vi "Get_Kinect_Depth_Array.vi"(8 "Index":i32, 9 "Far_Clip_Plane":u16=2040, 11 "Refnum_in":T1=refnum) -> (0 "2D_Array":u16[][](array[numeric]), 1 "1D_Array":u16[](array[numeric]), 2 "Image_out":T1, 3 "Refnum_out":T1)   [LabVIEW 2011]
uses:
  <vilib>/vision/Image Controls.llb/IMAQ Image.ctl
  Freenect Code/libfreenect.lvlib
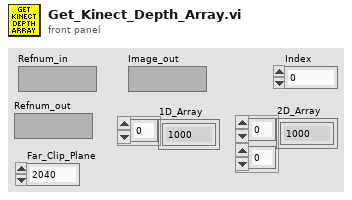
[diagram p1: front panel]
types:
  T1 = typedef "IMAQ Image.ctl" = refnum<image>
  T2 = enum16{"FREENECT_DEPTH_11BIT", "FREENECT_DEPTH_10BIT", "FREENECT_DEPTH_11BIT_PACKED", "FREENECT_DEPTH_10BIT_PACKED"}
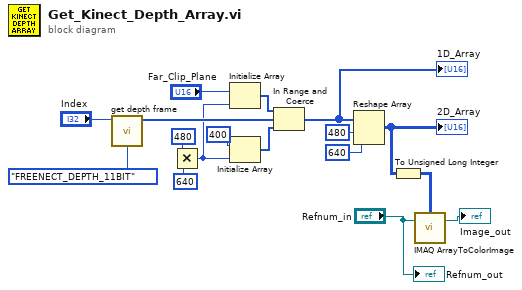
[diagram p0: block diagram]
diagram:
  n1 = call "get depth frame.vi"("fmt"=T2."FREENECT_DEPTH_11BIT", "index"="Index") -> ("Destination"=w11:u16[])  [unwired: 1 in, 8 out]
  n2 = Multiply(x=480, y=640) -> (x*y=w4:i32)
  n3 = Initialize Array("Far_Clip_Plane", w4) -> (w9:u16[])
  n4 = Initialize Array(u16 400 ("element"), w4) -> (w5:u16[])
  n5 = In Range and Coerce(upper limit=w9, x=w11, lower limit=w5) -> (coerced(x)=w12:u16[])  [unwired: 1 out]
  "1D_Array" <- w12
  n6 = Reshape Array(w12, 480 ("dimension size"), 640 ("dimension size")) -> (w1:u16[][])
  "2D_Array" <- w1
  n7 = To Unsigned Long Integer(number=w1) -> (unsigned 32bit integer=w2:u32[][])
  n8 = call "IMAQ ArrayToColorImage"("Image Pixels (U32)"=w2, "Image"="Refnum_in") -> ("Image Out"=→"Image_out":T1)  [unwired: 3 in, 1 out]
  "Refnum_out" <- "Refnum_in"
